vi "NI VeriStand - Save Configuration File (Path).vi"(8 "Error in":errorcluster, 10 "File Path":string, 11 "Runtime Configuration Ref in":refnum<k39>) -> (0 "Error out":errorcluster, 2 "Success":bool, 3 "Runtime Configuration Ref out":refnum<k39>)   [LabVIEW 2025, in "Runtime Configuration File API.lvlib"]
uses:
  Runtime Configuration File API.lvlib
  C:/NetCoreDLL/NationalInstruments.VeriStand.SystemDefinitionAPI.dll
  NetCoreDLL/NationalInstruments.VeriStand.SystemDefinitionAPI.dll
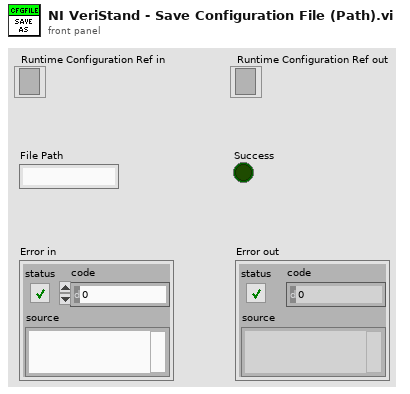
[diagram p1: front panel]
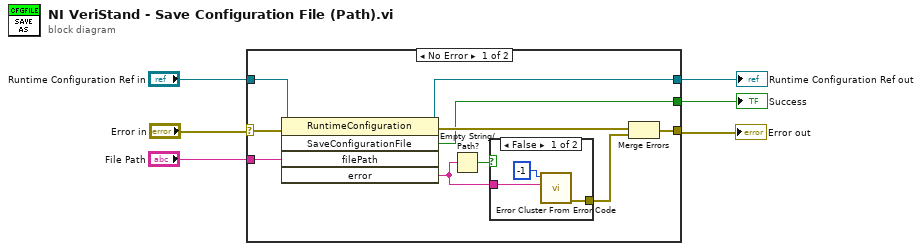
[diagram p0: block diagram]
diagram:
  n1 = case shown="No Error" "Error in" {
    selector: "Error in" -> [w16 _]
    tunnel: "Runtime Configuration Ref in" -> [w12 w20]
    tunnel: [w11 w20] -> w1
    tunnel: [w10 _] -> w2
    tunnel: [w14 _] -> w5
    tunnel: "File Path" -> [w8 _]
    frame No Error {
      n2 = invoke class="RuntimeConfiguration" method="SaveConfigurationFile"(reference=w12, error in=w16, "filePath"=w8) -> (reference out=w11:refnum<k39>, error out=w13:errorcluster, "SaveConfigurationFile"=w10:bool, "error"=w7:string)  [unwired: 2 in, 1 out]
      n3 = Empty String/Path?(string/path=w7) -> (empty?=w9:bool)
      n4 = case shown="False" w9 {
        tunnel: [w19 _] -> w15
        tunnel: w7 -> [w18 _]
        frame False {
          n5 = call <vilib>:"Error Cluster From Error Code.vi"("error message (\"\")"=w18, "error code (0)"=-1) -> ("error out"=w19:errorcluster)  [unwired: 7 in]
        }
        frame True {
        }
      }
      n6 = Merge Errors(w13, w15) -> (w14:errorcluster)
    }
    frame Error {
    }
  }
  "Runtime Configuration Ref out" <- w1
  "Success" <- w2
  "Error out" <- w5
